vi "Open Unflatten Refs.vi"(7 "App":refnum<vi>, 8 "error in (no error)":errorcluster, 10 "VI Path":path, 11 "LV-Protoc in":refnum<class "LV-Protoc.lvclass">) -> (0 "error out":errorcluster, 3 "LV-Protoc out":refnum<class "LV-Protoc.lvclass">, 5 "Unflatten Refs":T1)   [LabVIEW 2020, in "LV-Protoc.lvlib" / "LV-Protoc.lvclass"]
uses:
  LV-Protoc.lvclass
  Unflatten Refs.ctl
  <vilib>/Utility/traverseref.llb/TRef TravTarget.ctl
  Extract Field Terminal.ctl
  LV-Protoc.lvlib
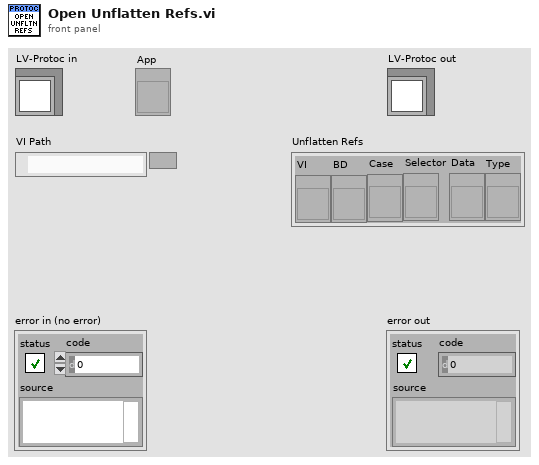
[diagram p1: front panel]
types:
  T1 = typedef "LV-Protoc.lvlib/Unflatten Refs.ctl" = cluster{"VI":refnum<vi>, "BD":refnum<vi>, "Case":refnum<vi>, "Selector":refnum<vi>, "Data":refnum<vi>, "Type":refnum<vi>}
  T2 = typedef "LV-Protoc.lvlib/Extract Field Terminal.ctl" = enum16{"NA 0", "NA 1", "Field Data", "Buffer", "NA 4", "Wire Type", "NA 6", "Field Number", "NA 8", "NA 9", "NA 10", "Buffer In"}
  T3 = typedef "TRef TravTarget.ctl" = enum16{"FP", "BD", "Other"}
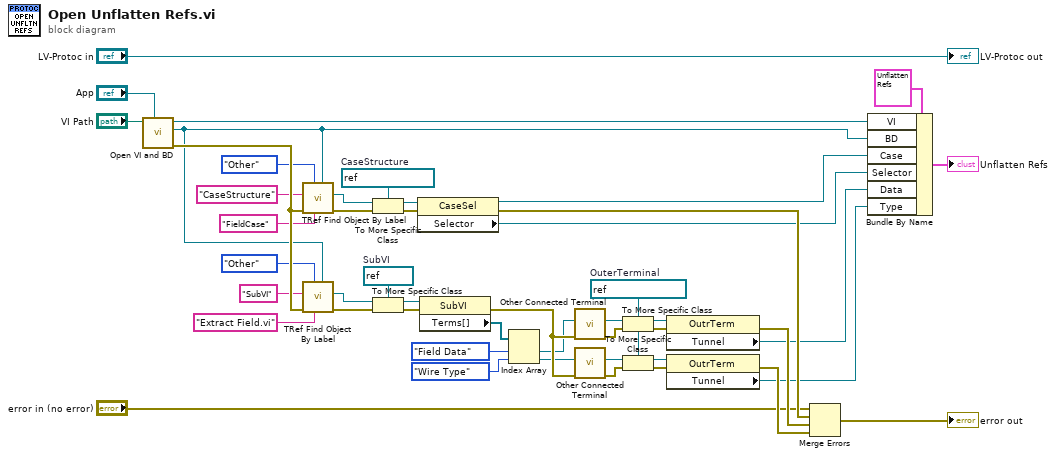
[diagram p0: block diagram]
diagram:
  w17 = refnum<vi> refnum  # OuterTerminal
  w34 = refnum<vi> refnum  # SubVI
  w31 = refnum<vi> refnum  # CaseStructure
  n1 = call "Open VI and BD.vi"("App"="App", "VI Path"="VI Path") -> ("error out"=w44:errorcluster, "BD"=w4:refnum<vi>, "VI"=w11:refnum<vi>)  [unwired: 7 in]
  n2 = call <vilib>:"TRef Find Object By Label.vi"("Other Refnum"=w4, "Label"="FieldCase", "Traverse Target"=TRef_TravTarget."Other", "error in (no error)"=w44, "Class Name"="CaseStructure") -> ("error out"=w33:errorcluster, "Found Obj Ref"=w32:refnum<vi>)  [unwired: 3 in, 2 out]
  n3 = call <vilib>:"TRef Find Object By Label.vi"("Other Refnum"=w4, "Label"="Extract Field.vi", "Traverse Target"=TRef_TravTarget."Other", "error in (no error)"=w44, "Class Name"="SubVI") -> ("error out"=w36:errorcluster, "Found Obj Ref"=w35:refnum<vi>)  [unwired: 3 in, 2 out]
  n4 = To More Specific Class(target class=w31, reference=w32, error in=w33) -> (specific class reference=w27:refnum<vi>, error out=w26:errorcluster)
  n5 = To More Specific Class(target class=w34, reference=w35, error in=w36) -> (specific class reference=w30:refnum<vi>, error out=w29:errorcluster)
  n6 = property class="CaseSel"(reference=w27, error in=w26) -> (reference out=w10:refnum<vi>, error out=w46:errorcluster, "Selector"=w9:refnum<vi>)
  n7 = property class="SubVI"(reference=w30, error in=w29) -> (error out=w45:errorcluster, "Terms[]"=w28:refnum<vi>[])  [unwired: 1 out]
  n8 = Index Array(array=w28, index #1=Extract_Field_Terminal."Field Data" ("Extract Field Terminal"), index #2=Extract_Field_Terminal."Wire Type" ("Extract Field Terminal")) -> (element #1=w23:refnum<vi>, element #2=w22:refnum<vi>)
  n9 = call "Other Connected Terminal.vi"("error in (no error)"=w45, "Terminal"=w23) -> ("error out"=w20:errorcluster, "Other"=w21:refnum<vi>)  [unwired: 8 in]
  n10 = call "Other Connected Terminal.vi"("error in (no error)"=w45, "Terminal"=w22) -> ("error out"=w18:errorcluster, "Other"=w19:refnum<vi>)  [unwired: 8 in]
  n11 = To More Specific Class(target class=w17, reference=w21, error in=w20) -> (specific class reference=w16:refnum<vi>, error out=w15:errorcluster)
  n12 = To More Specific Class(target class=w17, reference=w19, error in=w18) -> (specific class reference=w13:refnum<vi>, error out=w14:errorcluster)
  n13 = property class="OutrTerm"(reference=w16, error in=w15) -> (error out=w47:errorcluster, "Tunnel"=w8:refnum<vi>)  [unwired: 1 out]
  n14 = property class="OutrTerm"(reference=w13, error in=w14) -> (error out=w48:errorcluster, "Tunnel"=w7:refnum<vi>)  [unwired: 1 out]
  n15 = Merge Errors("error in (no error)", w46, w47, w48) -> (→"error out":errorcluster)
  n16 = Bundle By Name(cluster=T1 {"VI"=refnum, "BD"=refnum, "Case"=refnum, "Selector"=refnum, "Data"=refnum, "Type"=refnum} ("Unflatten Refs"), "VI"=w11, "BD"=w4, "Case"=w10, "Selector"=w9, "Data"=w8, "Type"=w7) -> (→"Unflatten Refs":T1)
  "LV-Protoc out" <- "LV-Protoc in"
